vi "CallRead.vi"(6 "Time out?":u8, 8 "error in (no error)":errorcluster, 11 "FPGA VI引用输入":refnum<k20>) -> (0 "error out":errorcluster, 2 "Data Out":u8, 3 "FPGA VI引用输出":refnum<k20>)   [LabVIEW 2013]
uses:
  <vilib>/rvi/interface/common/niFpgaWaitOnOcc.vi
  <vilib>/Utility/error.llb/Error Cluster From Error Code.vi
  <vilib>/rvi/errors/niLvFpgaAdjustHostInterfaceError.vi
  <vilib>/rvi/interface/nirviReadWriteControl/nirviReadWriteControl.xnode
  <vilib>/rvi/interface/Simulation/niFpgaSimulationCallBeginRW.vi
  NiFpgaLv.dll
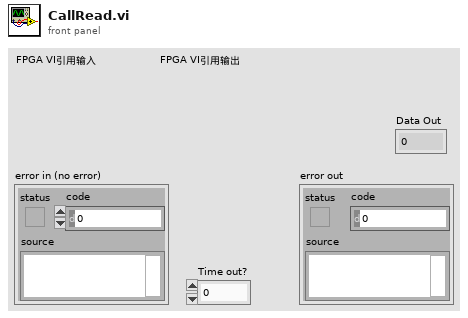
[diagram p1: front panel]
types:
  T1 = enum8{"IDLE", "SetIDLE", "Config", "Arm", "Read", "Write", "AutoRead"}
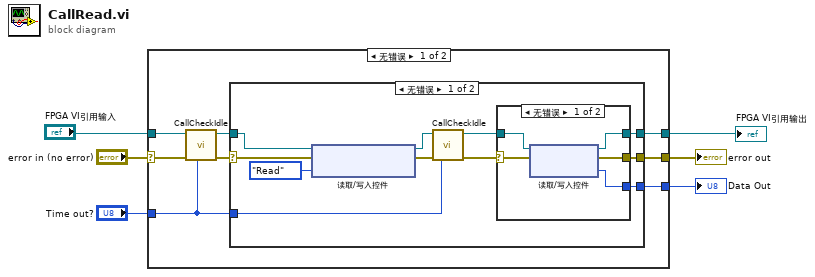
[diagram p0: block diagram]
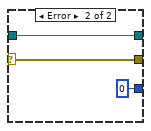
[diagram p2: hidden frame]
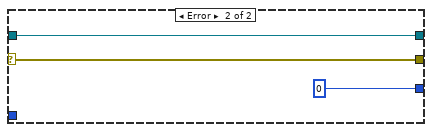
[diagram p3: hidden frame]
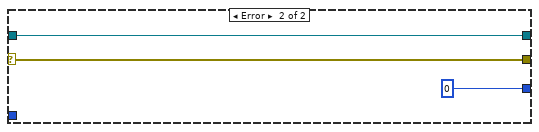
[diagram p4: hidden frame]
diagram:
  n1 = case shown="无错误" "error in (no error)" {
    selector: "error in (no error)" -> [w12 w39]
    tunnel: [w14 w39] -> w6
    tunnel: [w13 u8 0 ("I2C Protocol Output Data")] -> w5
    tunnel: "Time out?" -> [w11 _]
    tunnel: "FPGA VI引用输入" -> [w10 w37]
    tunnel: [w7 w37] -> w1
    frame No Error {
      n2 = call "CallCheckIdle.vi"("Time out?"=w11, "error in (no error)"=w12, "FPGA VI引用输入"=w10) -> ("error out"=w8:errorcluster, "FPGA VI引用输出"=w9:refnum<k20>)  [unwired: 7 in]
      n3 = case shown="无错误" w8 {
        selector: w8 -> [w23 w36]
        tunnel: [w25 u8 0 ("I2C Protocol Output Data 0")] -> w13
        tunnel: [w24 w36] -> w14
        tunnel: w11 -> [w19 _]
        tunnel: w9 -> [w22 w34]
        tunnel: [w15 w34] -> w7
        frame No Error {
          n4 = xnode "读取/写入控件"("FPGA VI引用输入"=w22, "错误输入"=w23, "ProtocolControl"=T1."Read") -> ("FPGA VI引用输出"=w18:refnum<k20>, "错误输出"=w21:errorcluster)
          n5 = call "CallCheckIdle.vi"("Time out?"=w19, "error in (no error)"=w21, "FPGA VI引用输入"=w18) -> ("error out"=w20:errorcluster, "FPGA VI引用输出"=w17:refnum<k20>)  [unwired: 7 in]
          n6 = case shown="无错误" w20 {
            selector: w20 -> [w28 w33]
            tunnel: [w27 u8 0 ("I2C Protocol Output Data 0")] -> w25
            tunnel: [w30 w33] -> w24
            tunnel: w17 -> [w29 w31]
            tunnel: [w26 w31] -> w15
            frame No Error {
              n7 = xnode "读取/写入控件"("FPGA VI引用输入"=w29, "错误输入"=w28) -> ("FPGA VI引用输出"=w26:refnum<k20>, "错误输出"=w30:errorcluster, "ReadData"=w27:u8)
            }
            frame Error {
            }
          }
        }
        frame Error {
        }
      }
    }
    frame Error {
    }
  }
  "Data Out" <- w5
  "error out" <- w6
  "FPGA VI引用输出" <- w1
